vi "Field Oriented Drive.vi"(8 "yaw angle":dbl, 9 "Xfield":dbl, 10 "Yfield":dbl) -> (1 "Xrobot":dbl, 2 "Yrobot":dbl)   [LabVIEW 2018]
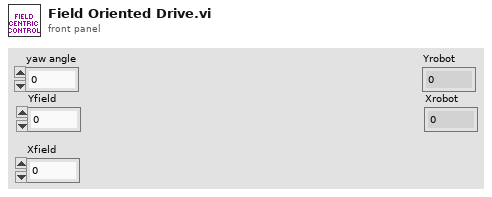
[diagram p1: front panel]
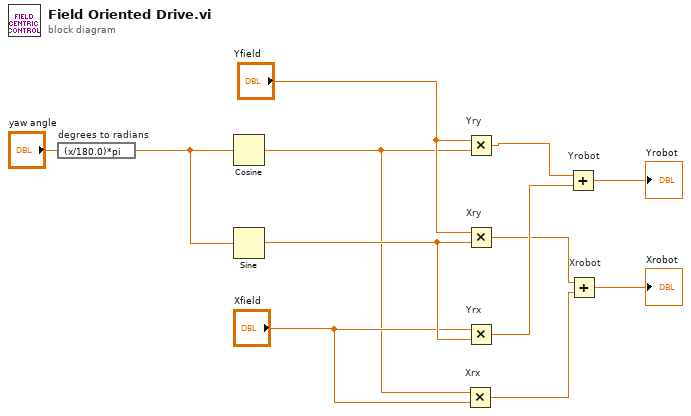
[diagram p0: block diagram]
diagram:
  n1 = expression code="(x/180.0)*pi" "degrees to radians"("yaw angle") -> (w11:dbl)
  n2 = Cosine(x=w11) -> (cos(x)=w7:dbl)
  n3 = Sine(x=w11) -> (sin(x)=w9:dbl)
  n4 = Multiply "Xrx"(x=w7, y="Xfield") -> (x*y=w3:dbl)
  n5 = Multiply "Yry"(x="Yfield", y=w7) -> (x*y=w5:dbl)
  n6 = Multiply "Xry"(x="Yfield", y=w9) -> (x*y=w4:dbl)
  n7 = Multiply "Yrx"(x="Xfield", y=w9) -> (x*y=w6:dbl)
  n8 = Add "Yrobot"(x=w5, y=w6) -> (x+y=→"Yrobot":dbl)
  n9 = Add "Xrobot"(x=w4, y=w3) -> (x+y=→"Xrobot":dbl)
